vi "WPI_CameraSetModeAttrMicroSoft.vi"(6 "Scaled":dbl, 7 "Attr Format":string="CameraAttributes::%s::Mode", 8 "error in":errorcluster, 9 "Value":string="Manual", 10 "Attr String":string, 11 "IMAQdx Session":T1) -> (0 "error out":errorcluster, 3 "IMAQdx Session out":T1)   [LabVIEW 2019]
doc: "Set the Mode of the attribute to Manual or Auto.\n\nThis software is licensed. Open the labview\\readme\\WPI Robotics Library Open Source License.txt file for more information."
uses:
  <resource>/objmgr/imaqdx.rc
  <vilib>/userDefined/High Color/IMAQdx.ctl
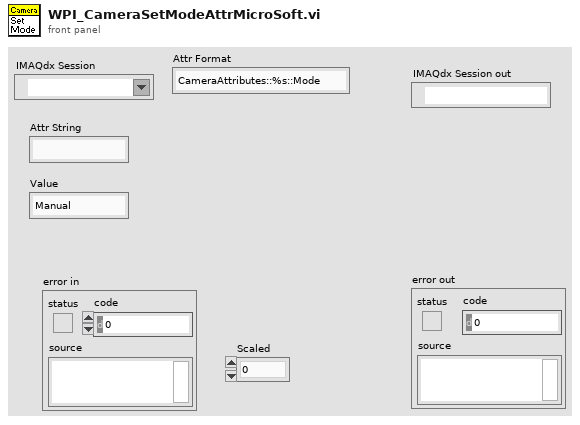
[diagram p1: front panel]
types:
  T1 = typedef "IMAQdx.ctl" = refnum<k21>
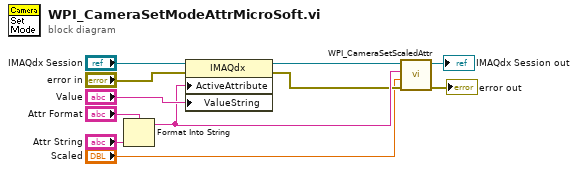
[diagram p0: block diagram]
diagram:
  n1 = Format Into String(format string="Attr Format", "Attr String") -> (resulting string=w4:string)  [unwired: 2 in, 1 out]
  n2 = property class="IMAQdx"(reference="IMAQdx Session", error in="error in", "ActiveAttribute"=w4, "ValueString"="Value") -> (reference out=w7:T1, error out=w3:errorcluster)
  n3 = call "WPI_CameraSetScaledAttr.vi"("error in (no error)"=w3, "Scaled"="Scaled", "Attr String"=w4, "Session In"=w7) -> ("error out"=→"error out":errorcluster, "IMAQdx Session"=→"IMAQdx Session out":T1)  [unwired: 6 in]
